vi "上传数据库.vi"(8 "错误输入":errorcluster) -> (0 "error out":errorcluster)   [LabVIEW 2017]
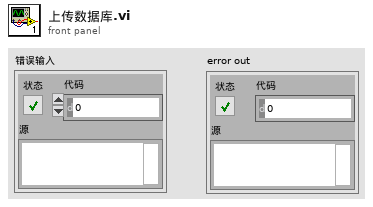
[diagram p1: front panel]
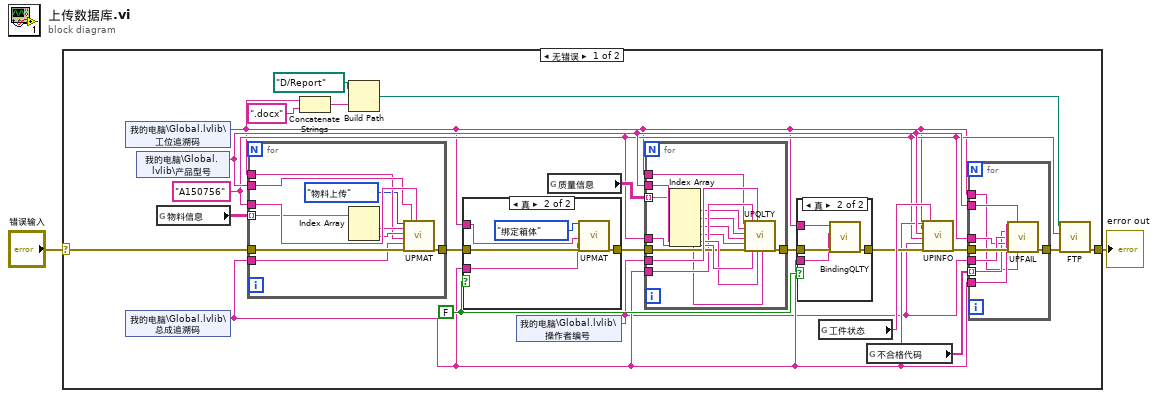
[diagram p0: block diagram]
diagram:
  n1 = case shown="无错误" "错误输入" {
    selector: "错误输入" -> [w16 w67]
    tunnel: [w21 w67] -> w2
    frame No Error {
      w22 = FALSE
      w5 = "A150756" ("产品型号")
      n2 = shared-variable "我的电脑\\Global.lvlib\\工位追溯码"() -> (w3:string)  [unwired: 1 in, 1 out]
      n3 = shared-variable "我的电脑\\Global.lvlib\\总成追溯码"() -> (w7:string)  [unwired: 1 in, 1 out]
      n4 = shared-variable "我的电脑\\Global.lvlib\\产品型号"() -> (w8:string)  [unwired: 1 in, 1 out]
      n5 = global read "追溯全部变量.vi" "物料信息"() -> (w15:string[][])
      n6 = for {
        tunnel: w5 -> [w66]
        tunnel: w8 -> [w65]
        tunnel: w16 -> [w64]
        tunnel: w15 -> [w63] mode=indexing
        tunnel: [w60] -> w24
        tunnel: w3 -> [w59]
        tunnel: w7 -> [w58]
        n7 = Index Array(array=w63) -> (element #1=w62:string, element #2=w61:string)  [unwired: 2 in]
        n8 = call "UPMAT.vi"("功能"=enum16{"物料上传", "绑定箱体"}."物料上传", "物料名称"=w62, "物料追溯码"=w61, "工位追溯码"=w59, "总成追溯码"=w58, "错误输入"=w64, "产品型号"=w65, "设备型号"=w66) -> ("错误输出"=w60:errorcluster)  [unwired: 10 in, 1 out]
      }
      n9 = Concatenate Strings(w3, ".docx" ("字符串")) -> (w18:string)
      n10 = Build Path(base path=path "D:/Report" ("基路径"), name or relative path=w18) -> (appended path=w17:path)
      n11 = case shown="真" w22 {
        tunnel: w24 -> [w51 w56]
        tunnel: [w51 w55] -> w23
        tunnel: w3 -> [_ w54]
        tunnel: w7 -> [_ w53]
        frame False {
        }
        frame True {
          n12 = call "UPMAT.vi"("功能"=enum16{"物料上传", "绑定箱体"}."绑定箱体", "工位追溯码"=w54, "总成追溯码"=w53, "错误输入"=w56) -> ("错误输出"=w55:errorcluster)  [unwired: 14 in, 1 out]
        }
      }
      n13 = shared-variable "我的电脑\\Global.lvlib\\操作者编号"() -> (w6:string)  [unwired: 1 in, 1 out]
      n14 = global read "追溯全部变量.vi" "质量信息"() -> (w14:string[][])
      n15 = for {
        tunnel: w6 -> [w50]
        tunnel: w5 -> [w49]
        tunnel: w8 -> [w48]
        tunnel: w23 -> [w47]
        tunnel: w7 -> [w46]
        tunnel: w3 -> [w45]
        tunnel: w14 -> [w44] mode=indexing
        tunnel: [w39] -> w12
        n16 = Index Array(array=w44) -> (element #1=w43:string, element #2=w42:string, element #3=w41:string, element #4=w40:string, element #5=w38:string)  [unwired: 5 in]
        n17 = call "UPQLTY.vi"("工位追溯码"=w45, "检测项目"=w43, "单位"=w42, "检测值"=w41, "检测结果"=w40, "错误输入"=w47, "总成追溯码"=w46, "设备编号"=w49, "操作员"=w50, "产品型号"=w48, "标准值"=w38) -> ("error out"=w39:errorcluster)  [unwired: 8 in]
      }
      n18 = case shown="真" w22 {
        tunnel: w12 -> [w33 w37]
        tunnel: [w33 w34] -> w11
        tunnel: w7 -> [_ w36]
        tunnel: w3 -> [_ w35]
        frame False {
        }
        frame True {
          n19 = call "BindingQLTY.vi"("错误输入"=w37, "总成追溯码"=w36, "工位追溯码"=w35) -> ("error out"=w34:errorcluster)  [unwired: 4 in]
        }
      }
      n20 = global read "追溯全部变量.vi" "工件状态"() -> (w13:string)
      n21 = global read "追溯全部变量.vi" "不合格代码"() -> (w4:string[])
      n22 = call "UPINFO.vi"("总成追溯码"=w7, "工位追溯码"=w3, "产品型号"=w8, "设备编号"=w5, "操作员"=w6, "error in (no error)"=w11, "加工状态"=w13) -> ("error out"=w10:errorcluster)  [unwired: 12 in]
      n23 = for {
        tunnel: w10 -> [w32]
        tunnel: [w31] -> w9
        tunnel: w8 -> [w30]
        tunnel: w7 -> [w29]
        tunnel: w6 -> [w28]
        tunnel: w5 -> [w27]
        tunnel: w4 -> [w26] mode=indexing
        tunnel: w3 -> [w25]
        n24 = call "UPFAIL.vi"("总成追溯码"=w29, "产品型号"=w30, "不合格代码"=w26, "操作员"=w28, "下线位置"=w27, "错误输入"=w32, "工位追溯码"=w25) -> ("错误输出"=w31:errorcluster)  [unwired: 8 in]
      }
      n25 = call "FTP.vi"("error in (no error)"=w9, "远程路径"=w5, "local path"=w17) -> ("error out"=w21:errorcluster)  [unwired: 8 in]
    }
    frame Error {
    }
  }
  "error out" <- w2
